vi "Subscribe.vi"(0 "STOMP in":refnum<class "STOMP.lvclass">, 1 "Destination":string, 2 "ack":T2, 3 "headers":T1[](array[typedef]), 5 "error in (no error)":errorcluster, 6 "Receipt?":bool=TRUE, 8 "ForceId":u64) -> (14 "STOMP out":refnum<class "STOMP.lvclass">, 16 "Subscription ID":u64, 19 "error out":errorcluster)   [LabVIEW 2017, in "STOMP.lvclass"]
uses:
  STOMP.lvclass
  Typedefs/Type_AckHeader.ctl
  Typedefs/Type_FrameHeader.ctl
  Typedefs/Type_ClientFrameType.ctl
  Typedefs/Type_ClientFrame.ctl
  Typedefs/Type_ActiveSubscription.ctl
  STOMP.lvclass/STOMP.ctl
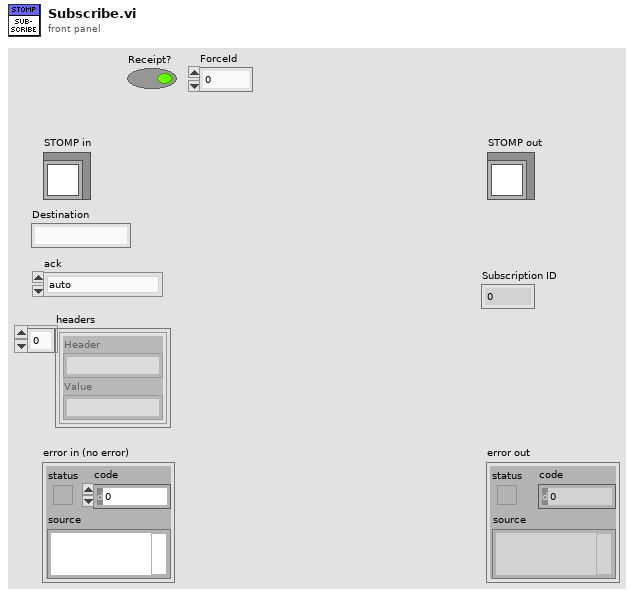
[diagram p1: front panel]
types:
  T1 = typedef "STOMP.lvclass/Type_FrameHeader.ctl" = cluster{"Header":string, "Value":string}
  T2 = typedef "STOMP.lvclass/Type_AckHeader.ctl" = enum16{"auto", "client", "client-individual"}
  T3 = typedef "STOMP.lvclass/Type_ActiveSubscription.ctl" = cluster{"id":u64, "receipt":bool, "Destination":string, "ack":T2, "headers":T1[]}
  T4 = typedef "STOMP.lvclass/Type_ClientFrame.ctl" = cluster{"Type":T5, "Headers":T1[], "Body":string}
  T5 = typedef "STOMP.lvclass/Type_ClientFrameType.ctl" = enum16{"Undefined", "SEND", "SUBSCRIBE", "UNSUBSCRIBE", "BEGIN", "COMMIT", "ABORT", "ACK", "NACK", "DISCONNECT"}
  T6 = typedef "LabVIEW STOMP.lvlib/STOMP.lvclass/ObjectAttributes.ctl" = cluster{"address":string, "port":u16, "ConnectionRef":refnum<k5>, "messageQueue":refnum<queue>, "receiptQueue":refnum<queue>, "errorQueue":refnum<queue>, "sendQueue":refnum<queue>, "currentReceiptNumber":u64, "currentSubscriptionId":u64, "closeConnection":bool, "activeSubscriptions":T7[]}
  T7 = typedef "Type_ActiveSubscription.ctl" = cluster{"id":u64, "receipt":bool, "Destination":string, "ack":T8, "headers":T9[]}
  T8 = typedef "Type_AckHeader.ctl" = enum16{"auto", "client", "client-individual"}
  T9 = typedef "LabVIEW STOMP.lvlib/STOMP.lvclass/Type_FrameHeader.ctl" = cluster{"Header":string, "Value":string}
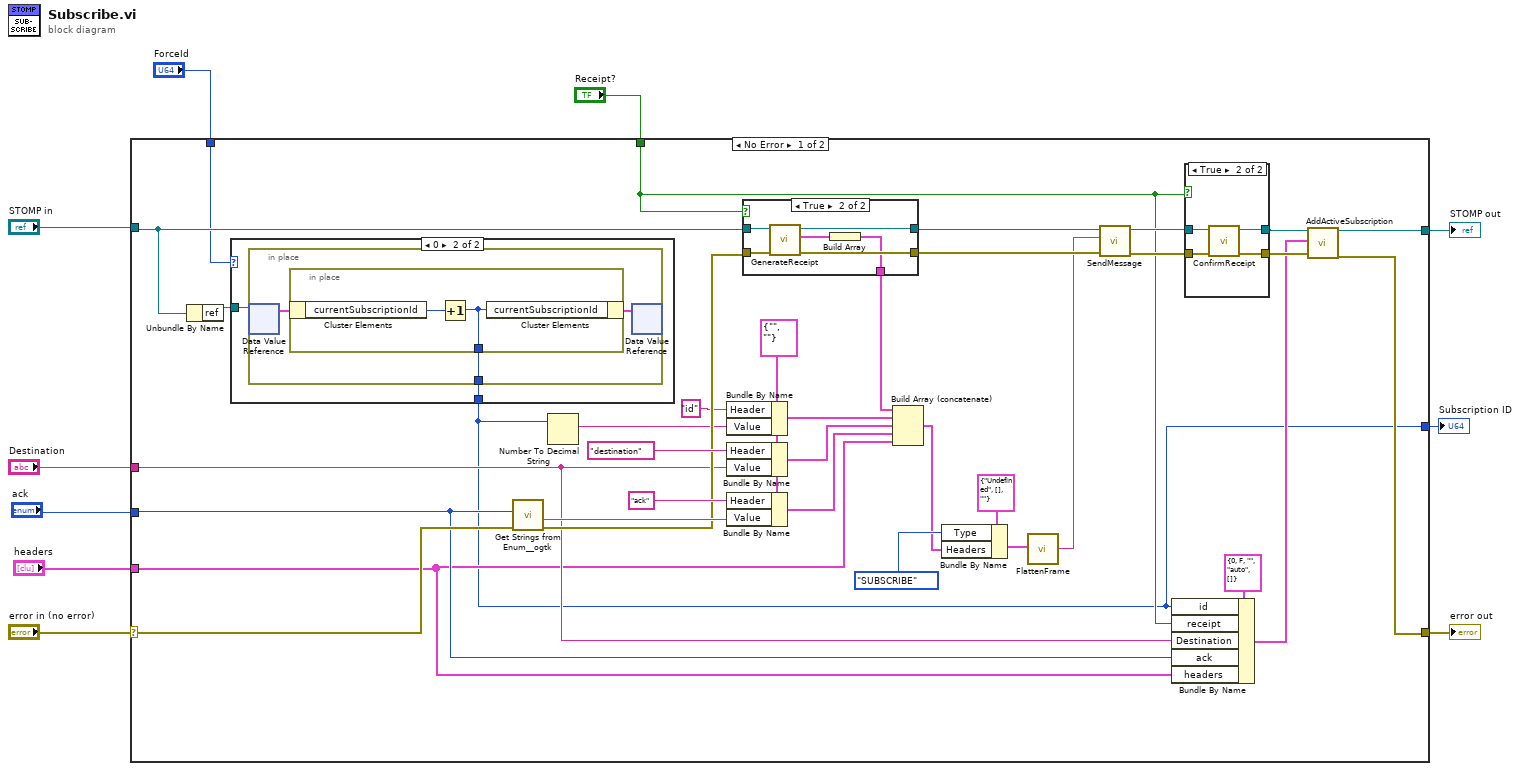
[diagram p0: block diagram]
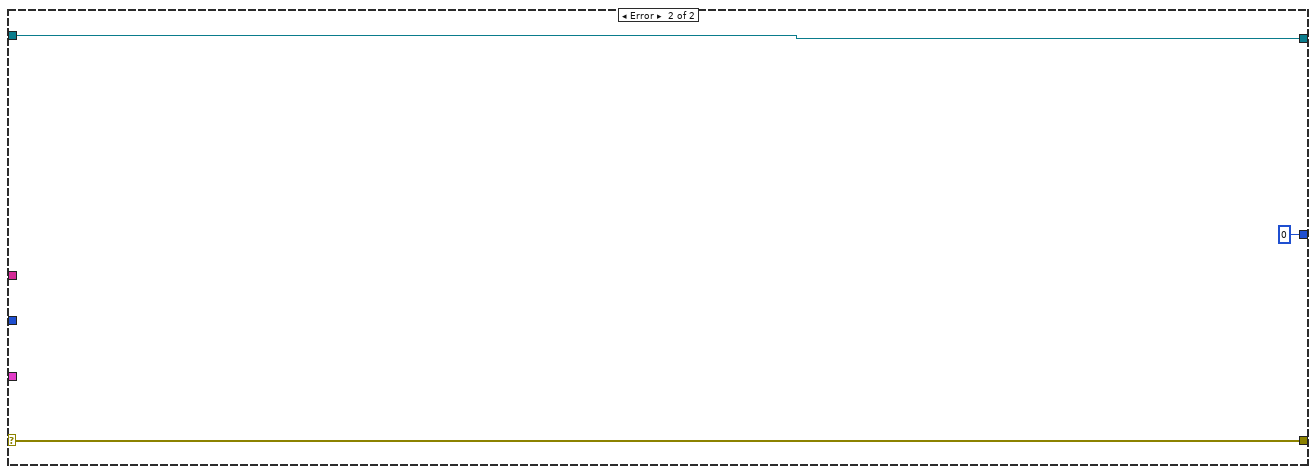
[diagram p5: hidden frame]
diagram:
  n1 = case shown="No Error" "error in (no error)" {
    selector: "error in (no error)" -> [w36 w70]
    tunnel: [w23 w70] -> w9
    tunnel: [w22 w69] -> w7
    tunnel: "STOMP in" -> [w27 w69]
    tunnel: "Destination" -> [w15 _]
    tunnel: "ack" -> [w14 _]
    tunnel: "Receipt?" -> [w16 _]
    tunnel: "headers" -> [w13 _]
    tunnel: "ForceId" -> [w12 _]
    tunnel: [w11 u64 0 ("ForceId")] -> w1
    frame No Error {
      w38 = T1 {"Header"="", "Value"=""}
      n2 = Unbundle By Name(w27) -> ("ref"=w28:refnum<data-value>)
      n3 = case shown="0" w12 {
        selector: w12 -> [w46 _]
        tunnel: [w46 w48] -> w11
        tunnel: w28 -> [_ w47]
        frame Default {
        }
        frame 0 {
          n4 = in-place {
            in-place-border: [w51] -> w48
            n5 = in-place-dvr #1(w47) -> (w50:T6)  [unwired: 1 out]
            n6 = in-place {
              in-place-border: [w52] -> w51
              n7 = in-place-cluster #2(w50) -> ("currentSubscriptionId"=w53:u64)
              n8 = Increment(x=w53) -> (x+1=w52:u64)
              n9 = in-place-cluster #2("currentSubscriptionId"=w52) -> (w49:T6)
            }
            n10 = in-place-dvr #1(w49) -> ()  [unwired: 2 out]
          }
        }
      }
      n11 = call <userlib>:"Get Strings from Enum__ogtk.vi"("error in (no error)"=w36, "Enum"=w14) -> ("error out"=w26:errorcluster, "String Value"=w35:string)  [unwired: 6 in, 2 out]
      n12 = Number To Decimal String(number=w11) -> (decimal integer string=w17:string)  [unwired: 1 in]
      n13 = Bundle By Name(cluster=w38, "Header"="id", "Value"=w17) -> (w40:T1)
      n14 = Bundle By Name(cluster=w38, "Header"="destination", "Value"=w15) -> (w39:T1)
      n15 = Bundle By Name(cluster=w38, "Header"="ack", "Value"=w35) -> (w34:T1)
      n16 = case shown="True" w16 {
        tunnel: w27 -> [w55 w61]
        tunnel: w26 -> [w54 w60]
        tunnel: [w55 w59] -> w29
        tunnel: [w54 w58] -> w30
        tunnel: [_ w56] -> w31
        frame False {
        }
        frame True {
          n17 = call-dynamic "GenerateReceipt.vi"("error in (no error)"=w60, "STOMP in"=w61) -> ("error out"=w58:errorcluster, "Receipt Header"=w57:T1, "STOMP out"=w59:refnum<class "STOMP.lvclass">)  [unwired: 7 in]
          n18 = Build Array(w57) -> (w56:T1[])
        }
      }
      n19 = Build Array (concatenate)(w31, w40, w39, w34, w13) -> (w42:T1[])
      n20 = Bundle By Name(cluster=T4 {"Type"=enum."Undefined", "Headers"=[], "Body"=""} ("Type_ClientFrame"), "Type"=Type_ClientFrameType."SUBSCRIBE", "Headers"=w42) -> (w41:T4)
      n21 = call "FlattenFrame.vi"("Client Frame"=w41) -> ("flattened frame"=w20:string)  [unwired: 18 in]
      n22 = call-dynamic "SendMessage.vi"("error in (no error)"=w30, "data in"=w20, "STOMP in"=w29) -> ("error out"=w32:errorcluster, "STOMP out"=w33:refnum<class "STOMP.lvclass">)  [unwired: 7 in]
      n23 = Bundle By Name(cluster=T3 {"id"=0, "receipt"=FALSE, "Destination"="", "ack"=enum."auto", "headers"=[]} ("activeSubscription"), "id"=w11, "receipt"=w16, "Destination"=w15, "ack"=w14, "headers"=w13) -> (w19:T3)
      n24 = case shown="True" w16 {
        tunnel: w33 -> [w62 w67]
        tunnel: w32 -> [w63 w66]
        tunnel: [w63 w65] -> w24
        tunnel: [w62 w64] -> w25
        frame False {
        }
        frame True {
          n25 = call-dynamic "ConfirmReceipt.vi"("error in (no error)"=w66, "STOMP in"=w67) -> ("error out"=w65:errorcluster, "STOMP out"=w64:refnum<class "STOMP.lvclass">)  [unwired: 8 in]
        }
      }
      n26 = call-dynamic "AddActiveSubscription.vi"("STOMP in"=w25, "activeSubscription"=w19, "error in (no error)"=w24) -> ("STOMP out"=w22:refnum<class "STOMP.lvclass">, "error out"=w23:errorcluster)  [unwired: 15 in]
    }
    frame Error {
    }
  }
  "error out" <- w9
  "STOMP out" <- w7
  "Subscription ID" <- w1
